vi "sub_RTCM-str_parsing.vi"(11 "RTCM recv-str":string) -> (2 "val":bool, 3 "RTCM arr":u8[](array[numeric]) format="%02x")   [LabVIEW 2019]
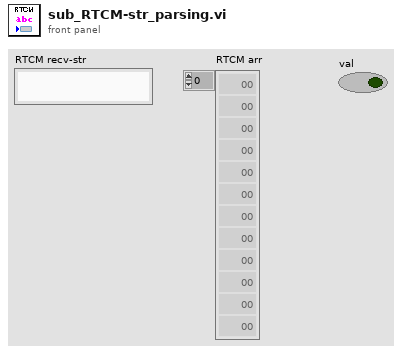
[diagram p1: front panel]
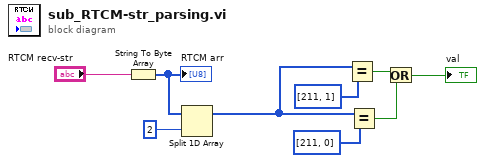
[diagram p0: block diagram]
diagram:
  n1 = String To Byte Array(string="RTCM recv-str") -> (unsigned byte array=w2:u8[])
  "RTCM arr" <- w2
  n2 = Split 1D Array(array=w2, index=2 ("인덱스")) -> (first subarray=w5:u8[])  [unwired: 1 out]
  n3 = Equal?(x=w5, y=u8[] [211, 1]) -> (x = y?=w7:bool)
  n4 = Equal?(x=w5, y=u8[] [211, 0]) -> (x = y?=w8:bool)
  n5 = Or(x=w7, y=w8) -> (x .or. y?=→"val":bool)
